vi "Update Channels.vi"(6 "Settings":T1={"Step Values"=[], "Only Execute When Test Running"=TRUE, "Reset Sequence When Test Starts"=TRUE, "Current Sequence ID"=0, "Total Iterations"=0, "Last Timestamp"=0.0, "Number of Sequence Steps"=0, "Num of Analog Channels"=0, "Num of Digital Channels"=0, "Delay Before Starting Sequence"=0.0, "Changed"=FALSE}, 8 "error in":errorcluster, 9 "Analog":bool, 10 "Previous Number of Channels":i32=8, 11 "Plugin in":refnum<class "Sequencer with Output Values.lvclass">) -> (0 "error out":errorcluster, 1 "Channels to Remove":string[](array[string]), 2 "Updated Number of Channels":i32, 3 "Plugin out":refnum<class "Sequencer with Output Values.lvclass">, 5 "Channels to Add":refnum<class "Producer Channel.lvclass">[](array[class]))   [LabVIEW 2020, in "Sequencer with Output Values.lvlib" / "Sequencer with Output Values.lvclass"]
uses:
  Sequencer with Output Values.lvclass
  Params.ctl
  Step Settings.ctl
  <vilib>/FlexLogger/SDK/PluginSDK.lvlibp/PEFClasses/SDK/Producer Channel/Producer Channel.lvclass
  <vilib>/FlexLogger/SDK/PluginSDK.lvlibp/PEFClasses/SDK/Channel/Data Type.ctl
  Global Strings.vi
  <vilib>/FlexLogger/SDK/PluginSDK.lvlibp/PEFClasses/SDK/Producer Channel/Create Producer Channel.vi
  <vilib>/FlexLogger/SDK/PluginSDK.lvlibp/PEFClasses/SDK/Plugin/Plugin.lvclass
  <vilib>/FlexLogger/SDK/PluginSDK.lvlibp
  <vilib>/FlexLogger/SDK/PluginSDK.lvlibp/PEFClasses/SDK/Channel/Channel.lvclass
  C:/Program Files/National Instruments/LabVIEW 2024/vi.lib/FlexLogger/SDK/PluginSDK.lvlibp/PEFClasses/SDK/Plugin/Plugin.lvclass
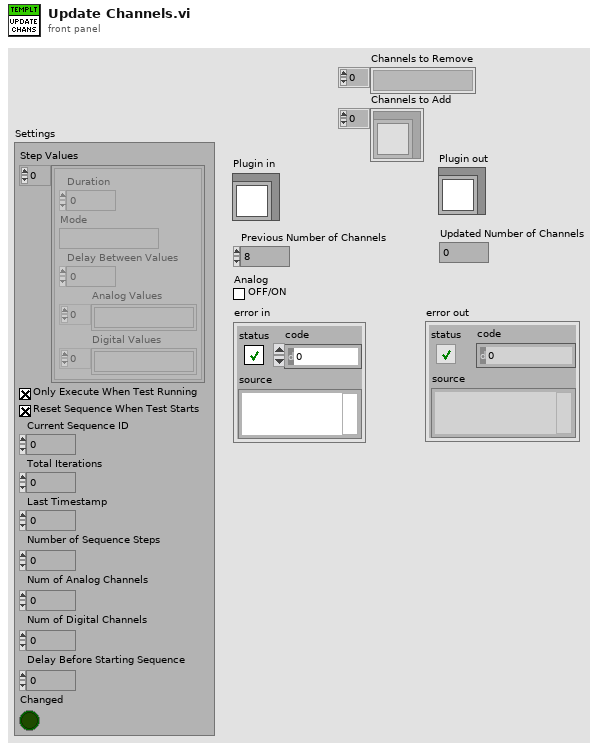
[diagram p1: front panel]
types:
  T1 = typedef "Sequencer with Output Values.lvlib/Sequencer with Output Values.lvclass/Params.ctl" = cluster{"Step Values":T2[], "Only Execute When Test Running":bool, "Reset Sequence When Test Starts":bool, "Current Sequence ID":u32, "Total Iterations":u32, "Last Timestamp":dbl, "Number of Sequence Steps":i32, "Num of Analog Channels":i32, "Num of Digital Channels":i32, "Delay Before Starting Sequence":dbl, "Changed":bool}
  T2 = typedef "Sequencer with Output Values.lvlib/Sequencer with Output Values.lvclass/Step Settings.ctl" = cluster{"Duration":dbl, "Mode":string, "Delay Between Values":dbl, "Analog Values":string[], "Digital Values":string[]}
  T3 = typedef "PluginSDK.lvlibp/Channel.lvclass/Data Type.ctl" = enum16{"Wfm (DBL)", "Wfm (Digital)"}
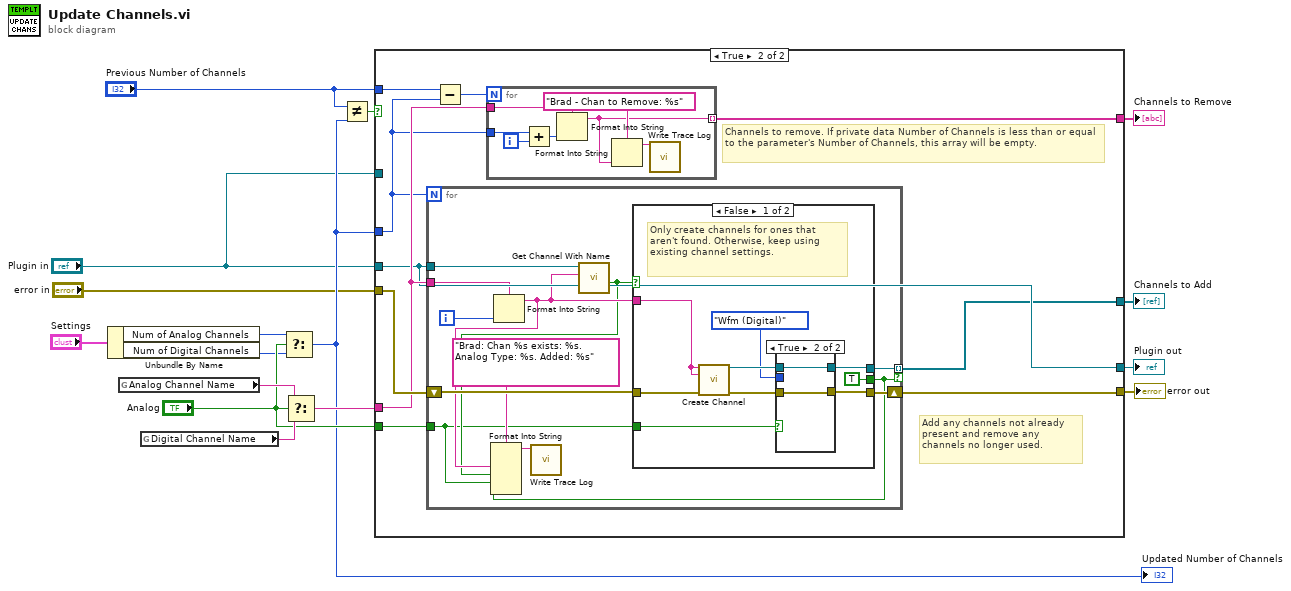
[diagram p0: block diagram]
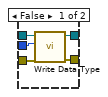
[diagram p3: hidden frame]
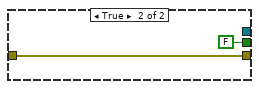
[diagram p4: hidden frame]
diagram:
  n1 = Unbundle By Name("Settings") -> ("Num of Analog Channels"=w4:i32, "Num of Digital Channels"=w3:i32)
  n2 = global read "Global Strings.vi" "Analog Channel Name"() -> (w14:string)
  n3 = global read "Global Strings.vi" "Digital Channel Name"() -> (w13:string)
  n4 = Select(t=w4, s="Analog", f=w3) -> (s? t:f=w8:i32)
  "Updated Number of Channels" <- w8
  n5 = Select(t=w14, s="Analog", f=w13) -> (s? t:f=w12:string)
  n6 = Not Equal?(x="Previous Number of Channels", y=w8) -> (x != y?=w16:bool)
  n7 = case shown="True" w16 {
    tunnel: "Previous Number of Channels" -> [_ w28]
    tunnel: w8 -> [_ w23]
    tunnel: "Plugin in" -> [w18 w20]
    tunnel: "error in" -> [w17 w26]
    tunnel: "Plugin in" -> [_ _]
    tunnel: [w18 w20] -> w11
    tunnel: [w17 w21] -> w10
    tunnel: w12 -> [_ w25]
    tunnel: "Analog" -> [_ w24]
    tunnel: [_ w22] -> w2
    tunnel: [_ w19] -> w1
    frame False {
    }
    frame True {
      # "Add any channels not already present and remove any channels no longer used."
      # "Channels to remove. If private data Number of Channels is less than or equal to the parameter's Number of Channels, this array will be empty."
      n8 = for {
        N: w23 -> [_]
        tunnel: w20 -> [w40]
        tunnel: [w39] -> w19 mode=indexing if=w29
        shift-right: [w38] -> w21
        shift-left: w26 -> [w37]
        tunnel: w25 -> [w36]
        tunnel: w24 -> [w30]
        i -> [w35]
        n9 = Format Into String(format string=w36, w35) -> (resulting string=w32:string)  [unwired: 2 in, 1 out]
        n10 = call <vilib>:"Get Channel With Name.vi"("Name"=w32, "Plugin in"=w40) -> ("Found?"=w31:bool)  [unwired: 7 in, 2 out]
        n11 = case shown="False" w31 {
          tunnel: w32 -> [w47 _]
          tunnel: [w42 _] -> w39
          tunnel: [TRUE FALSE] -> w29
          tunnel: [w41 w58] -> w38
          tunnel: w37 -> [w48 w58]
          tunnel: w30 -> [w46 _]
          frame False {
            # "Only create channels for ones that aren't found. Otherwise, keep using existing channel settings."
            n12 = call-poly <vilib>:"Create Channel.vi"("Unique Channel Identifier"=w47, "Default Channel Name"=w47, "error in (no error)"=w48) -> ("Producer Channel"=w45:refnum<class "Producer Channel.lvclass">, "error out"=w43:errorcluster)  [unwired: 11 in]
            n13 = case shown="True" w46 {
              tunnel: w45 -> [w54 w56]
              tunnel: Data_Type."Wfm (Digital)" ("Data Type") -> [w53 _]
              tunnel: w43 -> [w52 w55]
              tunnel: [w51 w56] -> w42
              tunnel: [w50 w55] -> w41
              frame False {
                n14 = call-dynamic "Write Data Type.vi"("error in (no error)"=w52, "Data Type"=w53, "Channel in"=w54) -> ("error out"=w50:errorcluster, "Channel out"=w51:refnum<class "Producer Channel.lvclass">)  [unwired: 7 in]
              }
              frame True {
              }
            }
          }
          frame True {
          }
        }
        n15 = Format Into String(format string="Brad: Chan %s exists: %s. Analog Type: %s. Added: %s", w32, w31, w30, w29) -> (resulting string=w33:string)  [unwired: 2 in, 1 out]
        n16 = call <vilib>:"Write Trace Log.vi"("Message"=w33) -> ()  [unwired: 10 in, 1 out]
      }
      n17 = Subtract(x=w28, y=w23) -> (x-y=w27:i32)
      n18 = for {
        N: w27 -> [_]
        tunnel: [w60] -> w22 mode=indexing
        tunnel: w23 -> [w64]
        tunnel: w25 -> [w62]
        i -> [w65]
        n19 = Add(x=w64, y=w65) -> (x+y=w63:i32)
        n20 = Format Into String(format string=w62, w63) -> (resulting string=w60:string)  [unwired: 2 in, 1 out]
        n21 = Format Into String(format string="Brad - Chan to Remove: %s", w60) -> (resulting string=w59:string)  [unwired: 2 in, 1 out]
        n22 = call <vilib>:"Write Trace Log.vi"("Message"=w59) -> ()  [unwired: 10 in, 1 out]
      }
    }
  }
  "Plugin out" <- w11
  "error out" <- w10
  "Channels to Remove" <- w2
  "Channels to Add" <- w1
